vi "interactive test top level driver.vi"() -> ()   [LabVIEW 2016, in "labssh_thijs.lvlib"]
uses:
  labssh_thijs.lvlib
panel:
  in  "Password":string="1234"
  in  "User Name":string="git"
  in  "Host Address":string="10.13.7.56"
  out "output":string="git\r\n"
  out "prompt before $ sign":string="git@hosman7dt3500-ubuntu:~"
  out "error out":errorcluster
  in  "input":string="whoami"
  in  "New Button":bool
  in  "OK Button":bool
  in  "Stop Button":bool=TRUE
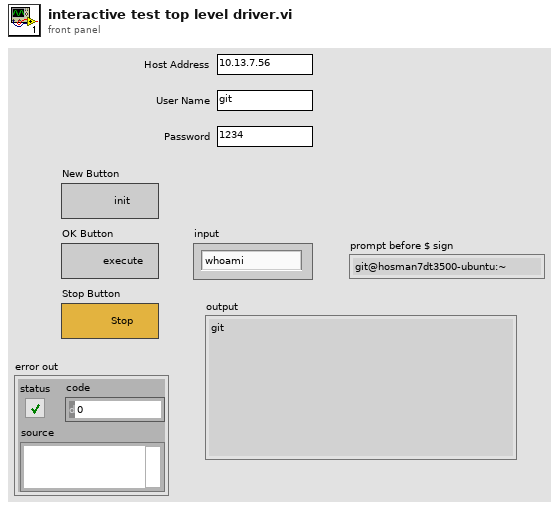
[diagram p1: front panel]
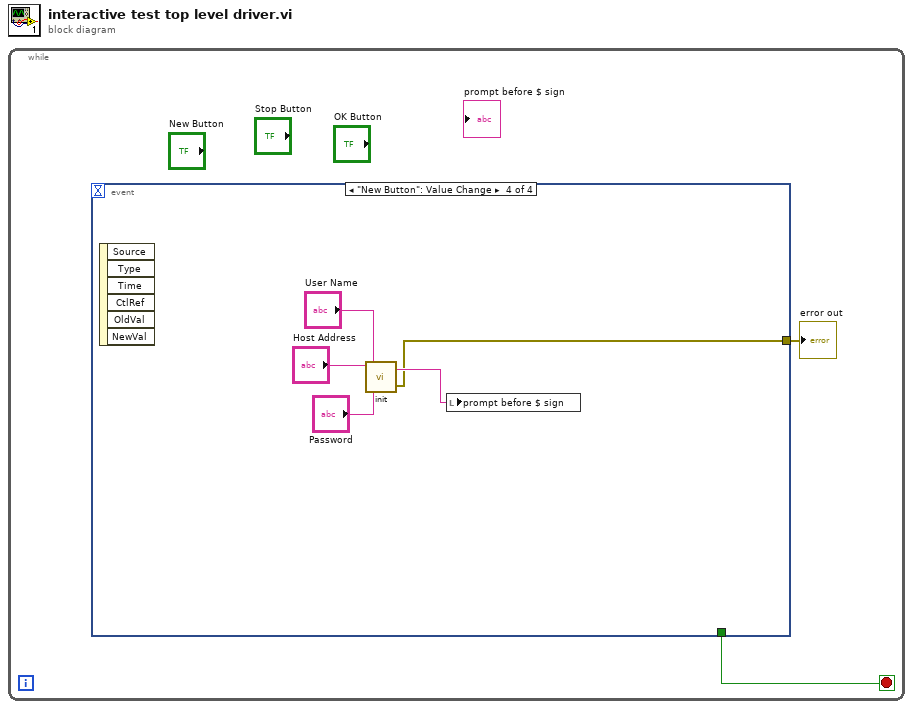
[diagram p0: block diagram]
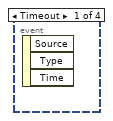
[diagram p2: hidden frame]
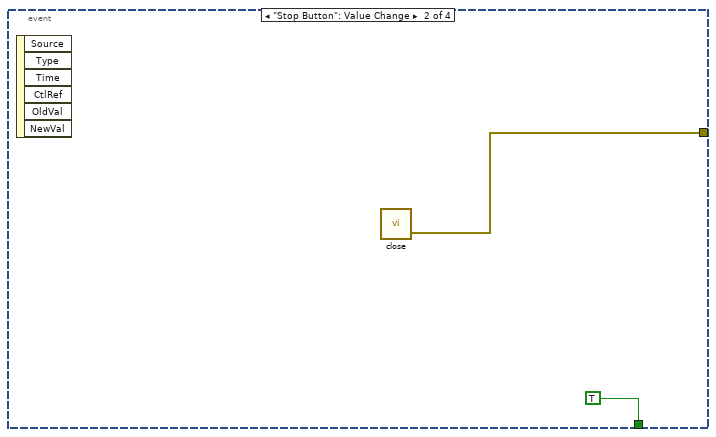
[diagram p3: hidden frame]
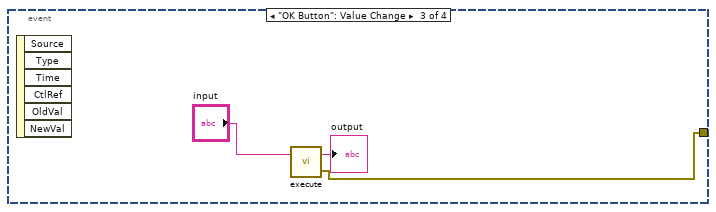
[diagram p4: hidden frame]
diagram:
  n1 = while {
    stop <- w2 stop-if-true
    n2 = event shown="[3] \"New Button\": Value Change" {
      selector: _ -> [_ _ _ _]
      dyn-events: _ -> [_ _ _ _]
      timeout: _ -> [_ _ _ _]
      tunnel: [_ TRUE _ _] -> w2
      tunnel: [_ w3 w5 w11] -> w1
      event Timeout {
        n3 = event-data() -> ()  [unwired: 1 in, 3 out]
      }
      event "Stop Button": Value Change {
        n4 = event-data() -> ()  [unwired: 1 in, 6 out]
        n5 = call "close.vi"() -> ("error out"=w3:errorcluster)  [unwired: 3 in]
      }
      event "OK Button": Value Change {
        n6 = event-data() -> ()  [unwired: 1 in, 6 out]
        n7 = call "execute.vi"("Input"="input") -> ("error out"=w5:errorcluster, "parsed reply"=→"output":string)  [unwired: 1 in]
      }
      event "New Button": Value Change {
        n8 = event-data() -> ()  [unwired: 1 in, 6 out]
        n9 = call "init.vi"("Password"="Password", "User Name"="User Name", "Host Address"="Host Address") -> ("error out"=w11:errorcluster, "prompt before $ sign"=w12:string)  [unwired: 1 in]
        n10 = local write "prompt before $ sign"(w12) -> ()
      }
    }
    "error out" <- w1
  }
